vi "WM Save Data.vi"(0 "Input Calibration":dbl format="%.2f", 1 "Input Offset":dbl format="%.2f", 2 "Input Data":dbl[][](array[numeric]) format="%.2f") -> ()   [LabVIEW 2012]
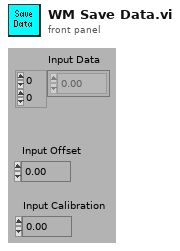
[diagram p1: front panel]
types:
  T1 = enum16{"open", "open or create", "create or replace", "create"}
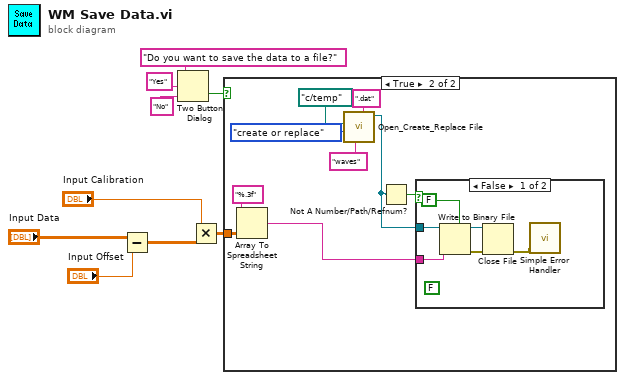
[diagram p0: block diagram]
diagram:
  n1 = Subtract(x="Input Data", y="Input Offset") -> (x-y=w5:dbl[][])
  n2 = Two Button Dialog(message="Do you want to save the data to a file?", 1:"No" ("F button name (\"Cancel\")"), 2:"Yes" ("T button name (\"OK\")")) -> (T button?=w6:bool)
  n3 = Multiply(x="Input Calibration", y=w5) -> (x*y=w4:dbl[][])
  n4 = case shown="True" w6 {
    tunnel: w4 -> [_ w17]
    frame False {
    }
    frame True {
      n5 = Array To Spreadsheet String(array=w17, 3:"%.3f" ("format string")) -> (spreadsheet string=w11:string)  [unwired: 1 in]
      n6 = call <vilib>:"Open_Create_Replace File.vi"("pattern"=".dat", "default name"="waves", "function (open:0)"=T1."create or replace", "start path  (Not A Path)"=path "c:/temp") -> ("refnum"=w10:refnum<file>)  [unwired: 4 in, 3 out]
      n7 = Not A Number/Path/Refnum?(number/path/refnum=w10) -> (NaN/Path/Refnum?=w12:bool)
      n8 = case shown="False" w12 {
        tunnel: w11 -> [w23 _]
        tunnel: w10 -> [w24 _]
        frame False {
          (unwired) FALSE ("append to file? (new file:F)")
          n9 = Write to Binary File(file (use dialog)=w24, data=w23, 5:FALSE ("prepend array or string size? (T)")) -> (refnum out=w22:refnum<file>, error out=w21:errorcluster)  [unwired: 3 in, 1 out]
          n10 = Close File(refnum=w22, error in=w21) -> (error out=w20:errorcluster)  [unwired: 1 out]
          n11 = call <vilib>:"Simple Error Handler.vi"("error in (no error)"=w20) -> ()  [unwired: 4 in, 5 out]
        }
        frame True {
        }
      }
    }
  }
